vi "Simulated PS Current.vi"() -> ()   [LabVIEW 2011, in "Simulated Beam VIs.lvlib"]
uses:
  Simulated Beam VIs.lvlib
panel:
  in  "Simulated PS Current":dbl[](array[numeric])
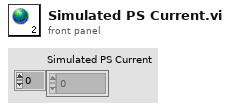
[diagram p1: front panel]
diagram:
